vi "Set Largest Decoration Visible.vi"(6 "Visible":bool, 8 "error in (no error)":errorcluster, 11 "VI Ref (calling VI)":refnum<vi>) -> (0 "error out":errorcluster, 3 "dup VI Ref":refnum<vi>)   [LabVIEW 2015, in "Utility.lvlib"]
uses:
  Utility.lvlib
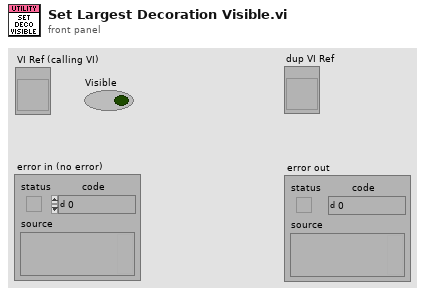
[diagram p1: front panel]
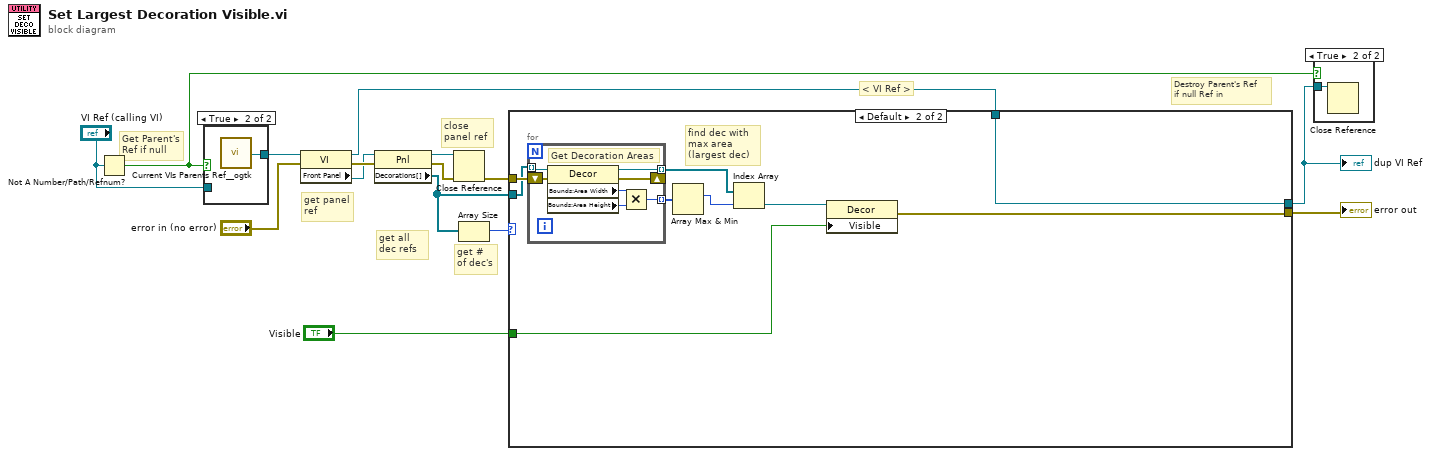
[diagram p0: block diagram]
diagram:
  # "Destroy Parent's Ref\nif null Ref in"
  # "Get Parent's\nRef if null"
  # "get # of dec's"
  # "get panel ref"
  # "get all dec refs"
  # "close panel ref"
  # "< VI Ref >"
  n1 = Not A Number/Path/Refnum?(number/path/refnum="VI Ref (calling VI)") -> (NaN/Path/Refnum?=w3:bool)
  n2 = case shown="True" w3 {
    tunnel: [w16 w17] -> w4
    tunnel: "VI Ref (calling VI)" -> [w16 _]
    frame False {
    }
    frame True {
      n3 = call <userlib>:"Current VIs Parents Ref__ogtk.vi"() -> ("Calling VI's Reference"=w17:refnum<vi>)  [unwired: 2 in]
    }
  }
  n4 = property on="Property Node" class="VI"(reference=w4, error in="error in (no error)") -> (reference out=w15:refnum<vi>, error out=w13:errorcluster, "Front Panel"=w10:refnum<vi>)
  n5 = property on="Property Node" class="Pnl"(reference=w10, error in=w13) -> (reference out=w14:refnum<vi>, error out=w12:errorcluster, "Decorations[]"=w7:refnum<vi>[])
  n6 = Close Reference(reference=w14, error in (no error)=w12) -> (error out=w9:errorcluster)
  n7 = Array Size(array=w7) -> (size(s)=w6:i32)
  n8 = case shown="Default" w6 {
    tunnel: w15 -> [w19 w22]
    tunnel: w9 -> [w18 w28]
    tunnel: [w18 w21] -> w8
    tunnel: [w19 w22] -> w2
    tunnel: w7 -> [_ w24]
    tunnel: "Visible" -> [_ w20]
    frame 0 {
      # "do nothing if no decorations"
    }
    frame Default {
      # "find dec with max area (largest dec)"
      n9 = for {
        tunnel: w24 -> [w35] mode=indexing
        tunnel: [w32] -> w27 mode=indexing
        shift-right: [w30] -> _
        shift-left: w28 -> [w31]
        tunnel: [w29] -> w25 mode=indexing
        # "Get Decoration Areas"
        n10 = property class="Decor"(reference=w35, error in=w31) -> (reference out=w29:refnum<vi>, error out=w30:errorcluster, "Bounds:Area Width"=w34:u32, "Bounds:Area Height"=w33:u32)
        n11 = Multiply(x=w34, y=w33) -> (x*y=w32:u32)
      }
      n12 = Array Max & Min(array=w27) -> (max index (indices)=w26:i32)  [unwired: 3 out]
      n13 = Index Array(array=w25, index=w26) -> (element=w23:refnum<vi>)
      n14 = property class="Decor"(reference=w23, "Visible"=w20) -> (error out=w21:errorcluster)  [unwired: 1 in, 1 out]
    }
  }
  "error out" <- w8
  "dup VI Ref" <- w2
  n15 = case shown="True" w3 {
    tunnel: w2 -> [_ w36]
    frame False {
    }
    frame True {
      n16 = Close Reference(reference=w36) -> ()  [unwired: 1 in, 1 out]
    }
  }
